vi "SPI Flash Erase Chip.vi"(10 "SPIIndex":i32, 11 "DevIndex":i32) -> (3 "function return":i32)   [LabVIEW 2010, in "usb2spi.lvlib"]
doc: "int WINAPI SPI_FlashEraseChip(int DevIndex,int SPIIndex);"
uses:
  usb2spi.lvlib
  USB2XXX.dll
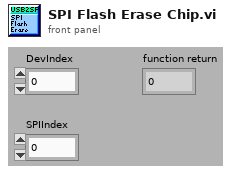
[diagram p1: front panel]
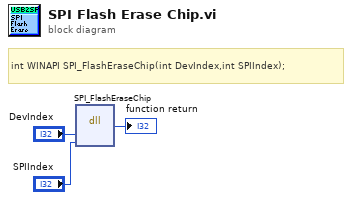
[diagram p0: block diagram]
diagram:
  # "int WINAPI SPI_FlashEraseChip(int DevIndex,int SPIIndex);"
  n1 = dll-call lib="G:/OtherWork/USB2XXX_Example/trunk/Labview/PublicFiles/usb2spi/USB2XXX.*" fn="SPI_FlashEraseChip"("DevIndex"="DevIndex", "SPIIndex"="SPIIndex") -> (→"function return":i32)  [unwired: 5 in, 2 out]
